vi "EditorPDF setPDFSubGraph.vi"(8 "error in (no error)":errorcluster, 11 "CreatePDF in":refnum<class "CreatePDF.lvclass">) -> (0 "error out":errorcluster, 3 "CreatePDF out":refnum<class "CreatePDF.lvclass">)   [LabVIEW 2018, in "CreatePDF.lvclass"]
uses:
  CreatePDF.lvclass
  CreatePDF.lvclass/CreatePDF.ctl
  Sub/EditorSub createPictureSub.vi
  <vilib>/Simplicity AI/SAI_PDF_API/Classes/Context/Methods/Public/Low Level/Add/SAI_PDF_Add Line Feed.vi
  <vilib>/Simplicity AI/SAI_PDF_API/Classes/Context/Context.lvclass
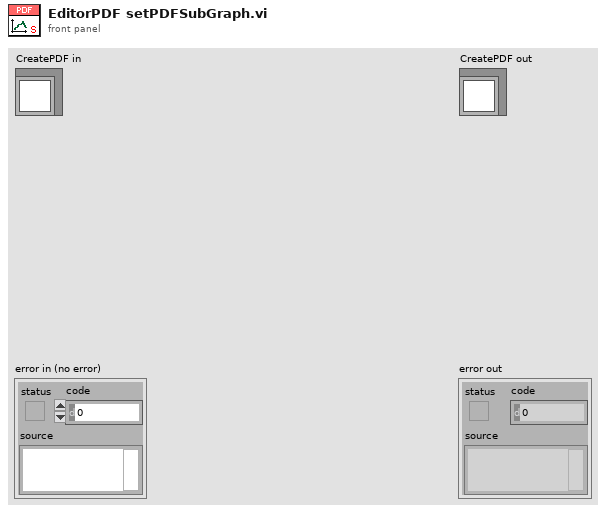
[diagram p1: front panel]
types:
  T1 = typedef "imagedata.ctl" = cluster{"image type":i32, "image depth":i32, "image":u8[], "mask":u8[], "colors":u32[], "Rectangle":cluster{"left":i16, "top":i16, "right":i16, "bottom":i16}}
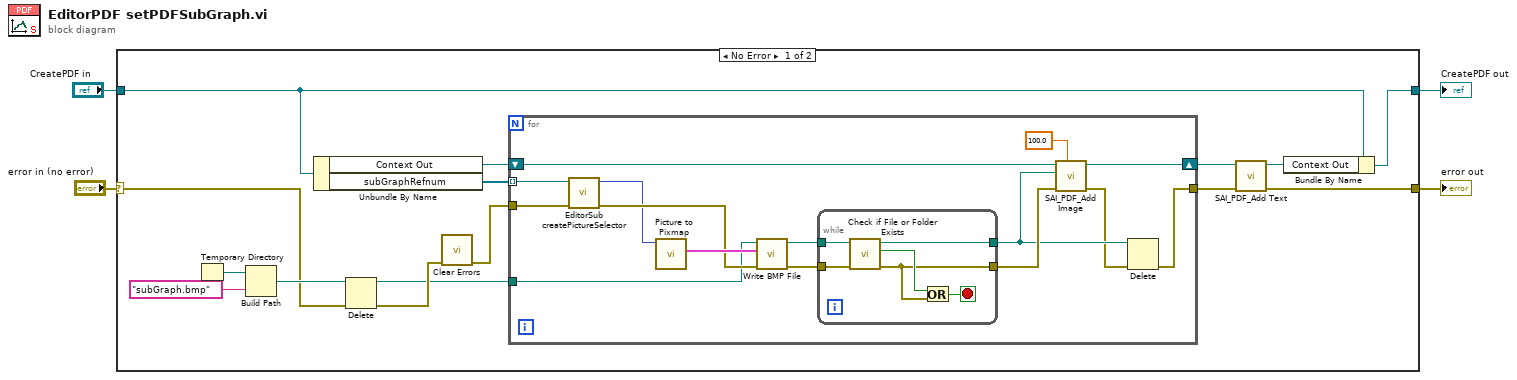
[diagram p0: block diagram]
diagram:
  n1 = case shown="No Error" "error in (no error)" {
    selector: "error in (no error)" -> [w10 w42]
    tunnel: [w6 w42] -> w2
    tunnel: [w18 w41] -> w1
    tunnel: "CreatePDF in" -> [w19 w41]
    frame No Error {
      n2 = Temporary Directory() -> (w15:path)
      n3 = Build Path(base path=w15, name or relative path="subGraph.bmp") -> (appended path=w13:path)
      n4 = Unbundle By Name(w19) -> ("Context Out"=w17:refnum<class "Context.lvclass">, "subGraphRefnum"=w16:refnum<vi>[])
      n5 = Delete(path (use dialog)=w13, error in=w10) -> (deleted path=w11:path, error out=w12:errorcluster)  [unwired: 4 out]
      n6 = call <vilib>:"Clear Errors.vi"("error in (no error)"=w12) -> ("error out"=w9:errorcluster)  [unwired: 5 in, 1 out]
      n7 = for {
        shift-right: [w28] -> w7
        shift-left: w17 -> [w29]
        tunnel: w16 -> [w24] mode=indexing
        tunnel: w11 -> [w23]
        tunnel: w9 -> [w27]
        tunnel: [w20] -> w8
        n8 = call-poly "EditorSub createPictureSelector.vi"("error in (no error)"=w27, "XY Graph"=w24) -> ("error out"=w26:errorcluster, "2D Picture"=w25:picture)  [unwired: 8 in]
        n9 = call <vilib>:"Picture to Pixmap.vi"("picture"=w25) -> ("image data"=w34:T1)  [unwired: 9 in, 1 out]
        n10 = call <vilib>:"Write BMP File.vi"("error in (no error)"=w26, "image data"=w34, "path to BMP file"=w23) -> ("error out"=w31:errorcluster, "path"=w32:path)  [unwired: 7 in]
        n11 = while {
          tunnel: w32 -> [w40]
          tunnel: w31 -> [w39]
          tunnel: [w36] -> w30
          tunnel: [w35] -> w22
          stop <- w37 stop-if-true
          n12 = call <vilib>:"Check if File or Folder Exists.vi"("error in (no error)"=w39, "path"=w40) -> ("error out"=w36:errorcluster, "file or folder exists?"=w38:bool, "dup path"=w35:path)  [unwired: 7 in]
          n13 = Or(x=w38, y=w36) -> (x .or. y?=w37:bool)
        }
        n14 = call <vilib>:"SAI_PDF_Add Image.vi"("Scale Percentage (100%)"=sgl 100.0, "error in"=w30, "File Name"=w22, "Context In"=w29) -> ("error out"=w21:errorcluster, "Context Out"=w28:refnum<class "Context.lvclass">)  [unwired: 2 in, 4 out]
        n15 = Delete(path (use dialog)=w22, error in=w21) -> (error out=w20:errorcluster)  [unwired: 5 out]
      }
      n16 = call-poly <vilib>:"SAI_PDF_Add Text.vi"("error in"=w8, "Context In"=w7) -> ("error out"=w6:errorcluster, "Context Out"=w5:refnum<class "Context.lvclass">)  [unwired: 2 in, 6 out]
      n17 = Bundle By Name(cluster=w19, "Context Out"=w5) -> (w18:refnum<class "CreatePDF.lvclass">)
    }
    frame Error {
    }
  }
  "error out" <- w2
  "CreatePDF out" <- w1
